vi "Configure Histogram Limits.vi"(6 "Histogram Right Limit (400E-6 s)":dbl=0.0004, 7 "Histogram Left Limit (-400E-6 s)":dbl=-0.0004, 8 "error in (no error)":errorcluster, 9 "Histogram Bottom Limit (-15.0 V)":dbl=-15.0, 10 "Histogram Top Limit (15.0 V)":dbl=15.0, 11 "VISA resource name":refnum<visa-resource-name>) -> (0 "error out":errorcluster, 3 "VISA resource name out":refnum<visa-resource-name>)   [LabVIEW 2016, in "Agilent 2000 3000 X-Series.lvlib"]
doc: "Configures the histogram limits that defines the area to be analyzed with the histogram.\n\n<b>Note:</b>\nThis VI is specific to the 6000-X Series oscilloscopes. These features are not available on other models."
uses:
  Agilent 2000 3000 X-Series.lvlib
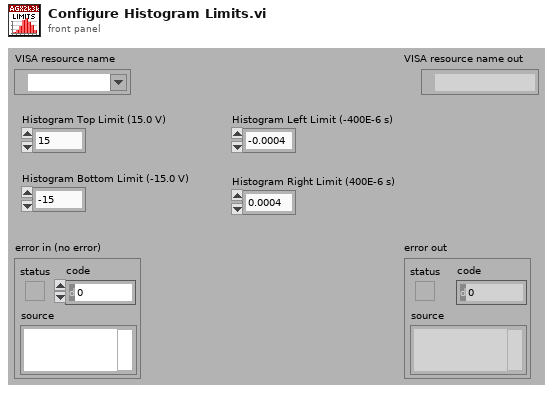
[diagram p1: front panel]
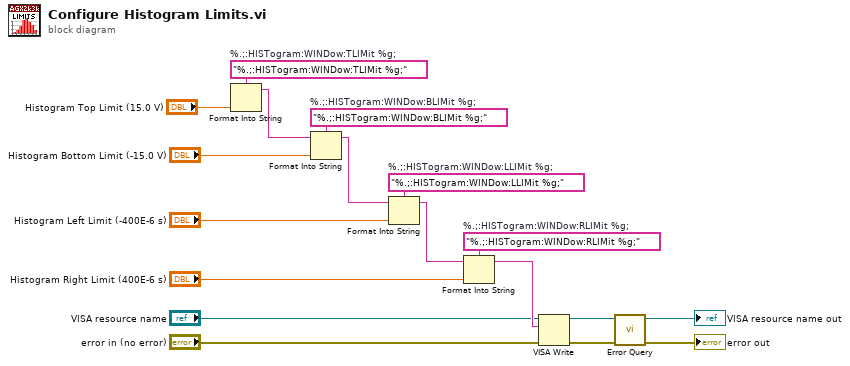
[diagram p0: block diagram]
diagram:
  w11 = "%.;:HISTogram:WINDow:RLIMit %g;"  # %.;:HISTogram:WINDow:RLIMit %g;
  w14 = "%.;:HISTogram:WINDow:LLIMit %g;"  # %.;:HISTogram:WINDow:LLIMit %g;
  w16 = "%.;:HISTogram:WINDow:TLIMit %g;"  # %.;:HISTogram:WINDow:TLIMit %g;
  w18 = "%.;:HISTogram:WINDow:BLIMit %g;"  # %.;:HISTogram:WINDow:BLIMit %g;
  n1 = Format Into String(format string=w16, "Histogram Top Limit (15.0 V)") -> (resulting string=w6:string)  [unwired: 2 in, 1 out]
  n2 = Format Into String(format string=w18, initial string=w6, "Histogram Bottom Limit (-15.0 V)") -> (resulting string=w5:string)  [unwired: 1 in, 1 out]
  n3 = Format Into String(format string=w14, initial string=w5, "Histogram Left Limit (-400E-6 s)") -> (resulting string=w12:string)  [unwired: 1 in, 1 out]
  n4 = Format Into String(format string=w11, initial string=w12, "Histogram Right Limit (400E-6 s)") -> (resulting string=w9:string)  [unwired: 1 in, 1 out]
  n5 = VISA Write(VISA resource name="VISA resource name", write buffer=w9, error in (no error)="error in (no error)") -> (VISA resource name out=w4:refnum<visa-resource-name>, error out=w3:errorcluster)  [unwired: 1 out]
  n6 = call "Error Query.vi"("error in (no error)"=w3, "VISA resource name"=w4) -> ("error out"=→"error out":errorcluster, "VISA resource name out"=→"VISA resource name out":refnum<visa-resource-name>)  [unwired: 6 in, 2 out]
